vi "capex read and process 4-20mA.vi"(7 "DAQmx Device Name":tag="cDAQ1Mod1", 8 "error in":errorcluster, 10 "Command":enum16{"Init", "read", "Close"}(ring)=enum."read", 11 "task in":refnum<k21>) -> (0 "error out":errorcluster, 2 "data":waveform(dbl)[](array[waveform]), 3 "task out":refnum<k21>)   [LabVIEW 2013]
uses:
  <vilib>/DAQmx/read.llb/DAQmx Read (Analog 1D Wfm NChan NSamp).vi
  <vilib>/DAQmx/configure/timing.llb/DAQmx Timing (Sample Clock).vi
  <vilib>/DAQmx/create/channels.llb/DAQmx Create Channel (AI-Current-Basic).vi
  <vilib>/DAQmx/miscellaneous.llb/DAQmx Fill In Error Info.vi
  <resource>/objmgr/daqmx.rc
panel:
  in  "Num of Channels (8)":i32=8
  in  "DAQNum":i32
  in  "Channel names":string[][](array[string])
  in  "new task name":string="I1"
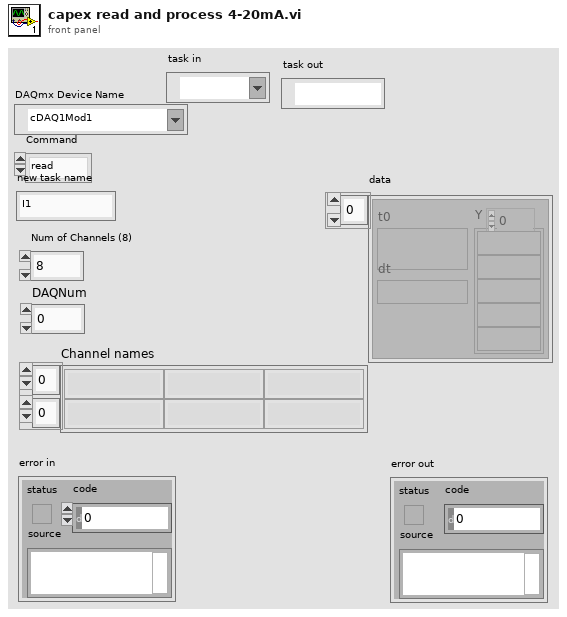
[diagram p1: front panel]
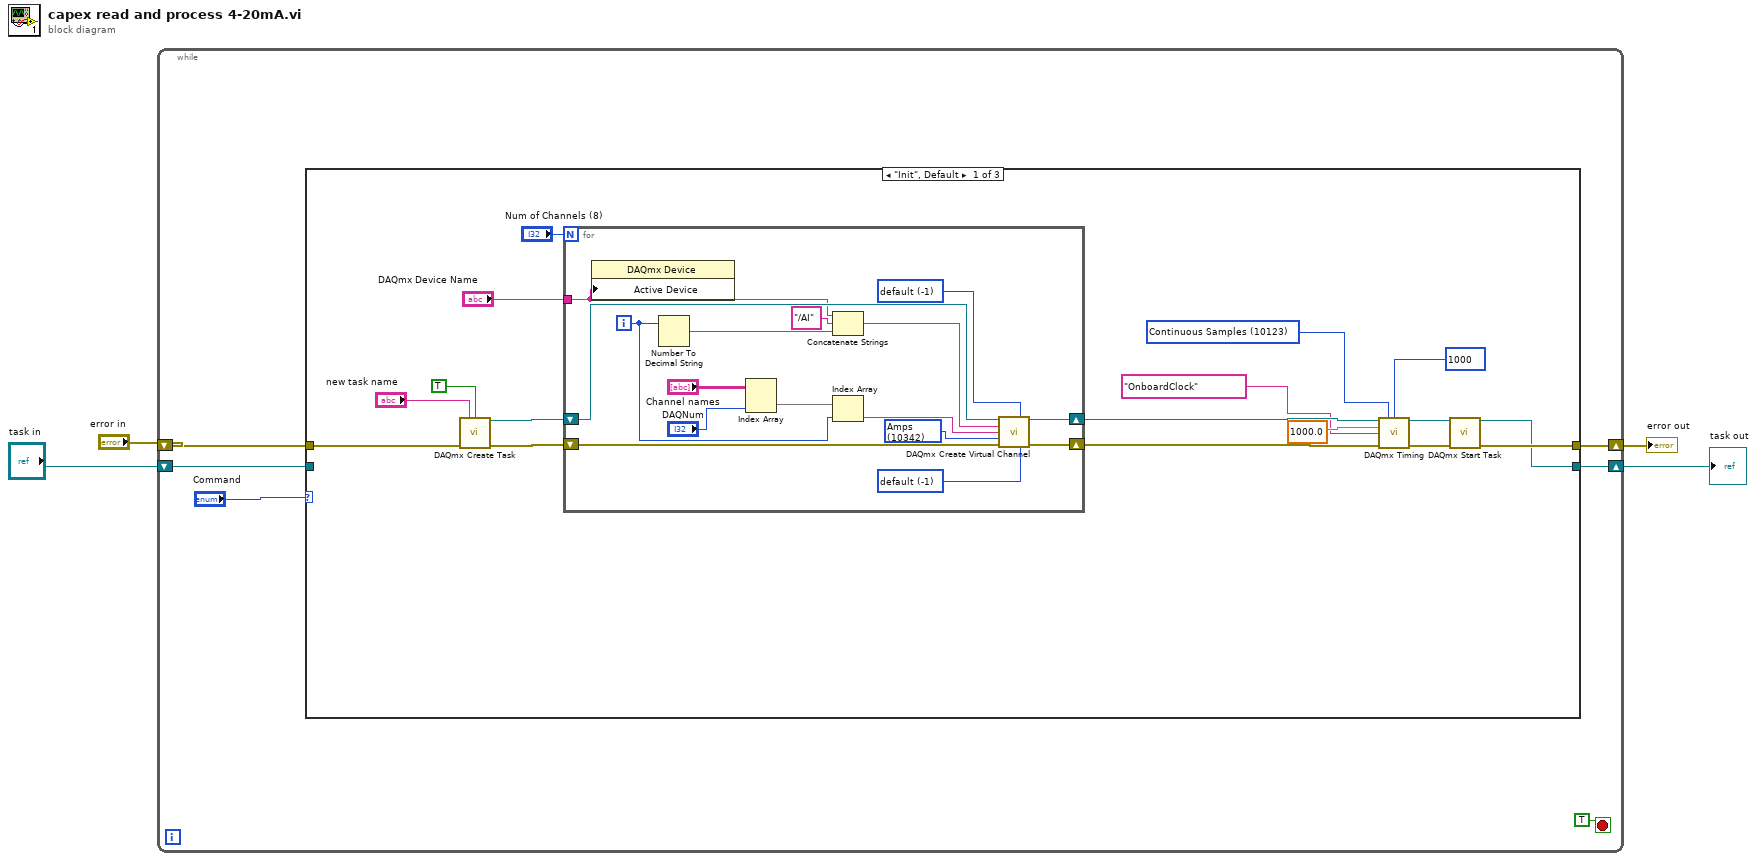
[diagram p0: block diagram]
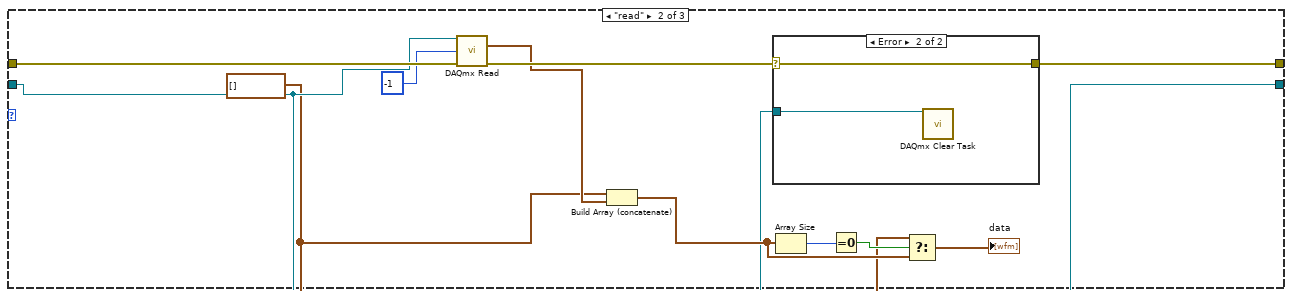
[diagram p2: hidden frame]
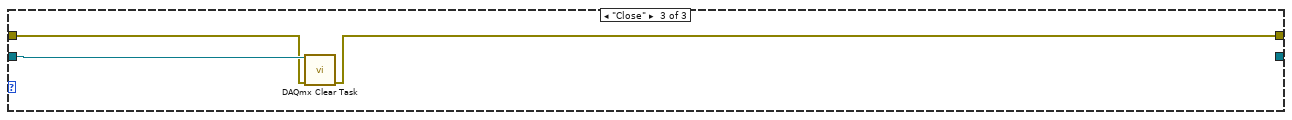
[diagram p4: hidden frame]
diagram:
  n1 = while {
    shift-right: [w9] -> w4
    shift-left: "error in" -> [w8]
    shift-right: [w5] -> w2
    shift-left: "task in" -> [w6]
    stop <- TRUE stop-if-true
    n2 = case shown="\"Init\", Default" "Command" {
      tunnel: [w12 w47 w58] -> w9
      tunnel: w8 -> [w27 w54 w59]
      tunnel: [w11 w48 _] -> w5
      tunnel: w6 -> [_ w48 w60]
      frame "Init", Default {
        w20 = 10123 items=["Finite Samples"=10178, "Continuous Samples"=10123, "Hardware Timed Single Point"=12522] ("sample mode")
        n3 = call <vilib>:"DAQmx Create Task.vi"("new task name"="new task name", "auto cleanup"=TRUE, "error in"=w27) -> ("task out"=w24:refnum<k21>, "error out"=w25:errorcluster)  [unwired: 11 in]
        n4 = for {
          N: "Num of Channels (8)" -> [_]
          shift-right: [w41] -> w18
          shift-left: w24 -> [w42]
          shift-right: [w40] -> w17
          shift-left: w25 -> [w43]
          tunnel: "DAQmx Device Name" -> [w35]
          i -> [w31]
          w36 = -1 items=["default"=-1, "Internal"=10200, "External"=10167] ("shunt resistor location")
          w37 = -1 items=["default"=-1, "RSE"=10083, "NRSE"=10078, "Differential"=10106, "Pseudodifferential"=12529] ("input terminal configuration")
          w38 = 10342 items=["Amps"=10342, "From Custom Scale"=10065] ("units")
          n5 = property class="DAQmx Device"("Active Device"=w35) -> ()  [unwired: 2 in, 2 out]
          n6 = Number To Decimal String(number=w31) -> (decimal integer string=w33:string)  [unwired: 1 in]
          n7 = Index Array(array="Channel names", index (col)="DAQNum") -> (element=w28:string[])  [unwired: 1 in]
          n8 = Concatenate Strings(w35, "/AI" ("string"), w33) -> (w39:string)
          n9 = Index Array(array=w28, index=w31) -> (element=w32:string)
          n10 = call-poly <vilib>:"DAQmx Create Virtual Channel.vi"("task in"=w42, "input terminal configuration"=w37, "physical channels"=w39, "name to assign"=w32, "units"=w38, "error in"=w43, "shunt resistor location"=w36) -> ("task out"=w41:refnum<k21>, "error out"=w40:errorcluster)  [unwired: 7 in]
        }
        n11 = call-poly <vilib>:"DAQmx Timing.vi"("task/channels in"=w18, "sample mode"=w20, "samples per channel"=1000, "rate"=1000.0, "source"=tag "OnboardClock", "error in"=w17) -> ("task out"=w14:refnum<k21>, "error out"=w13:errorcluster)  [unwired: 8 in]
        n12 = call <vilib>:"DAQmx Start Task.vi"("task/channels in"=w14, "error in"=w13) -> ("task out"=w11:refnum<k21>, "error out"=w12:errorcluster)  [unwired: 12 in]
      }
      frame "read" {
        w44 = waveform(dbl)[] []
        n13 = call-poly <vilib>:"DAQmx Read.vi"("task/channels in"=w48, "number of samples per channel"=-1, "error in"=w54) -> ("data"=w45:waveform(dbl)[], "error out"=w49:errorcluster)  [unwired: 10 in, 1 out]
        n14 = Build Array (concatenate)(w44, w45) -> (w51:waveform(dbl)[])
        n15 = case shown="Error" w49 {
          selector: w49 -> [w55 w56]
          tunnel: w48 -> [_ w57]
          tunnel: [w55 w56] -> w47
          frame No Error {
          }
          frame Error {
            n16 = call <vilib>:"DAQmx Clear Task.vi"("task in"=w57) -> ()  [unwired: 14 in, 1 out]
          }
        }
        n17 = Array Size(array=w51) -> (size(s)=w53:i32)
        n18 = Equal To 0?(x=w53) -> (x = 0?=w52:bool)
        n19 = Select(t=w44, s=w52, f=w51) -> (s? t:f=→"data":waveform(dbl)[])
      }
      frame "Close" {
        n20 = call <vilib>:"DAQmx Clear Task.vi"("task in"=w60, "error in"=w59) -> ("error out"=w58:errorcluster)  [unwired: 13 in]
      }
    }
  }
  "error out" <- w4
  "task out" <- w2
